vi "novasource_control.vi"(5 "Modulation Gain 2^i (i = -10 to 13)":i32 min=-10 max=13 step=1, 6 "Modulation On?":bool=TRUE, 7 "Frequency (1200-2000 MHz)":dbl=1251.451 min=1200.0 max=2000.0 step=0.001 format="%_7g") -> (0 "error out":errorcluster={"status"=FALSE, "code"=1073676294, "source"="VISA Read in novasource_control.vi"}, 1 "Locked?":bool=TRUE, 2 "RF State":bool=TRUE, 3 "Power":bool=TRUE)   [LabVIEW 2013]
uses:
  <vilib>/Instr/_visa.llb/VISA Configure Serial Port (Instr).vi
panel:
  in  "Case Constant\n(See Context Help)":i32
  out "Actual Gain":i32=1
  in  "Triggering Mode":u16(ring) items=["Continuous", "Momentary", "Toggle"]
  in  "Modulation Source":u16(ring)=1 items=["Internal Mod", "External Mod"]
  in  "Triggering Source":u16(ring) items=["Internal", "External"]
  in  "Attenuation Level (0-30)":i32 min=0 max=30 step=1
  in  "delay before read (ms)":u32=100
  in  "flow control":u16(ring) items=["None"=0, "XON/XOFF"=1, "RTS/CTS"=2, "DTR/DSR"=4]
  in  "stop bits":u16(ring)=10 items=["1.0"=10, "1.5"=15, "2.0"=20]
  in  "parity":u16(ring) items=["None", "Odd", "Even", "Mark", "Space"]
  in  "data bits":u16=8 min=5 max=8 step=1
  out "bytes read":u32=7
  in  "VISA resource name":refnum<visa-resource-name>="COM1"
  in  "baud rate":u32=38400
  # "Serial Settings"
  # "Nova Source Settings"
  # "Triggering"
  # "Modulation"
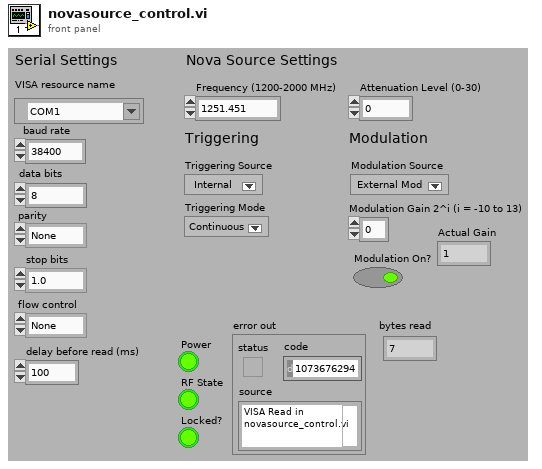
[diagram p1: front panel]
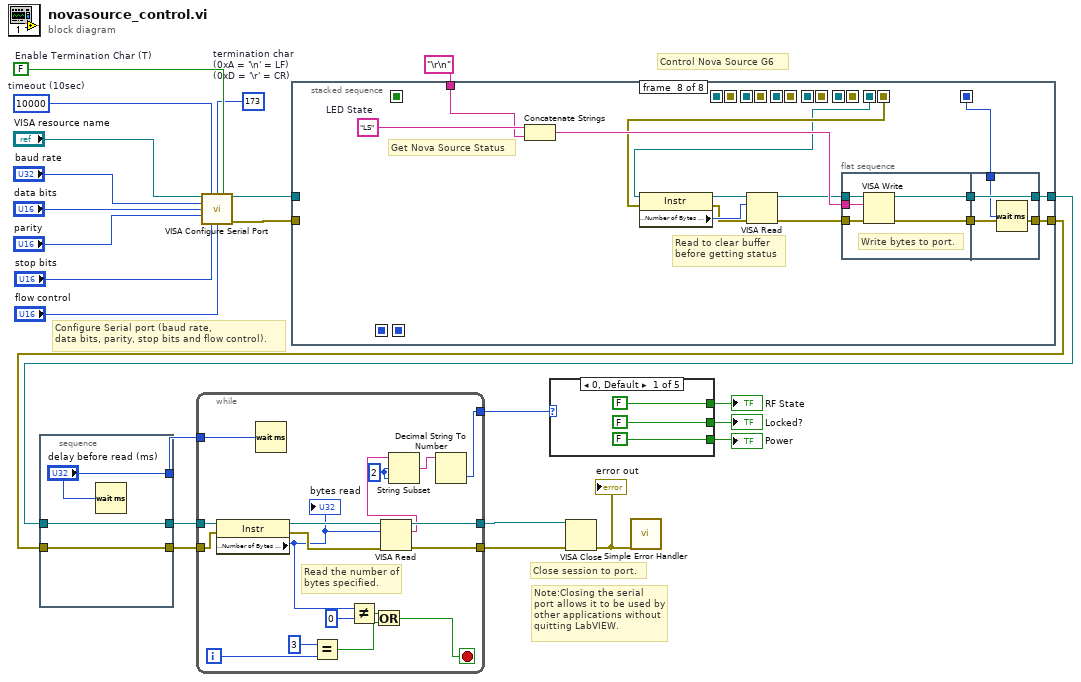
[diagram p0: block diagram]
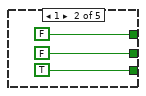
[diagram p2: hidden frame]
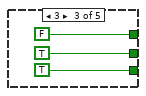
[diagram p3: hidden frame]
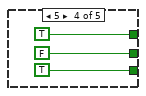
[diagram p4: hidden frame]
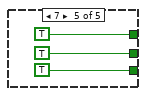
[diagram p5: hidden frame]
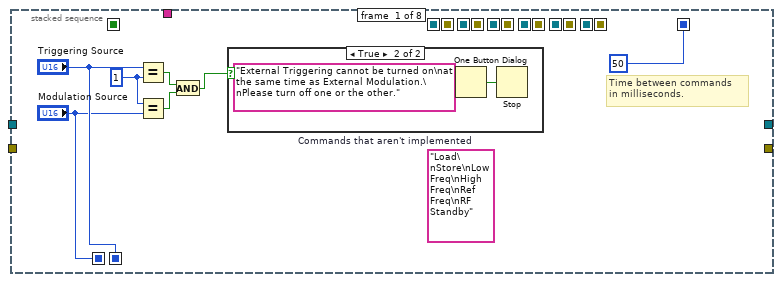
[diagram p6: hidden frame]
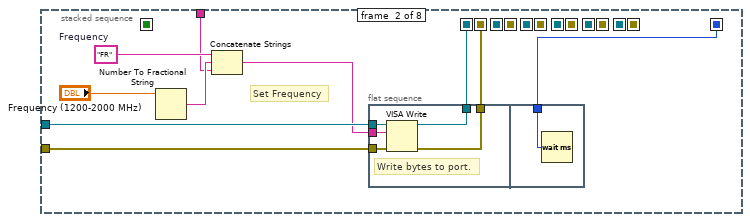
[diagram p8: hidden frame]
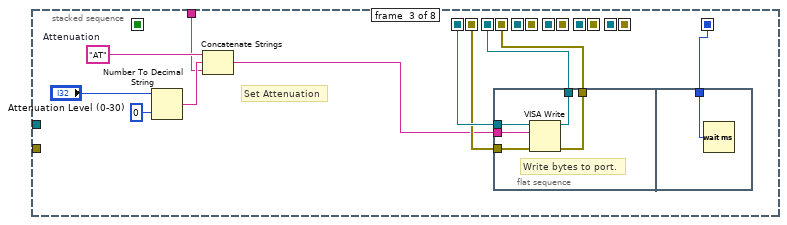
[diagram p9: hidden frame]
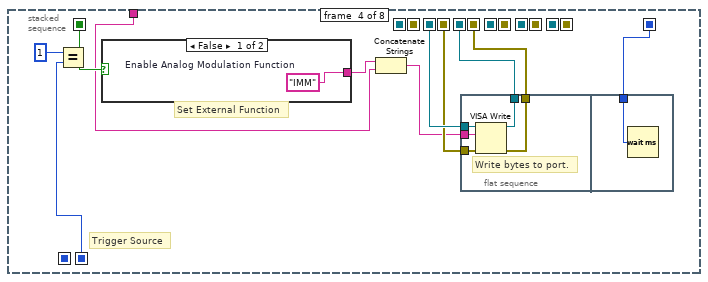
[diagram p10: hidden frame]
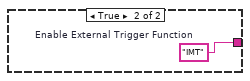
[diagram p11: hidden frame]
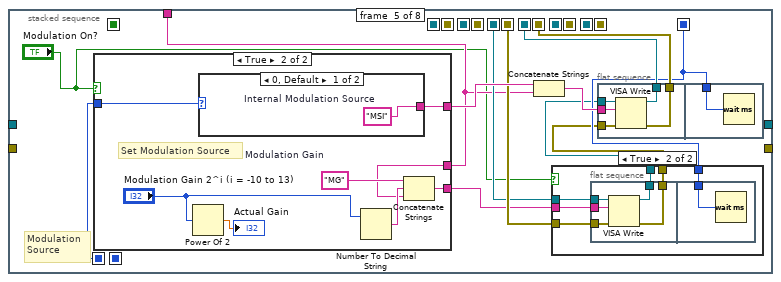
[diagram p12: hidden frame]
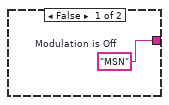
[diagram p14: hidden frame]
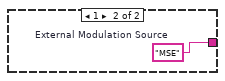
[diagram p15: hidden frame]
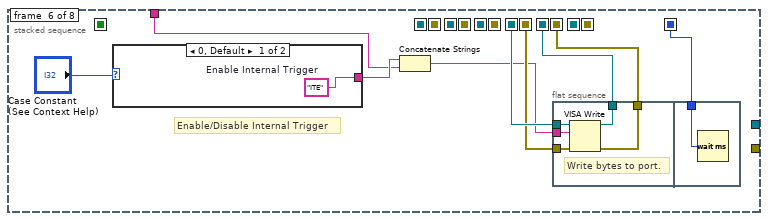
[diagram p16: hidden frame]
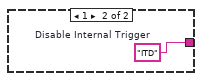
[diagram p17: hidden frame]
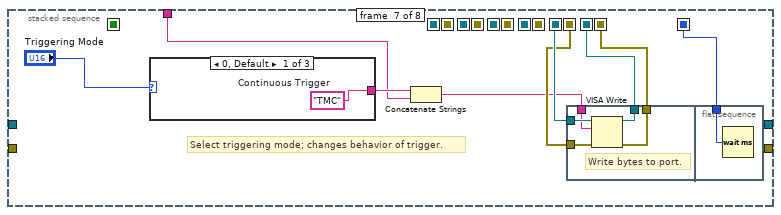
[diagram p18: hidden frame]
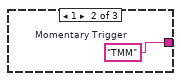
[diagram p19: hidden frame]
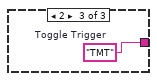
[diagram p20: hidden frame]
diagram:
  w10 = u8 173  # termination char (0xA = '\n' = LF) (0xD = '\r' = CR)
  w17 = FALSE  # Enable Termination Char (T)
  w18 = u32 10000  # timeout (10sec)
  # "Control Nova Source G6"
  # "Note:Closing the serial port allows it to be used by other applications without\nquitting LabVIEW."
  # "Configure Serial port (baud rate,\ndata bits, parity, stop bits and flow control)."
  # "Close session to port."
  n1 = call-poly "VISA Configure Serial Port"("VISA resource name"="VISA resource name", "timeout (10sec)"=w18, "termination char\n(0xA = '\\n' = LF)"=w10, "Enable Termination\nChar (T)"=w17, "baud rate (9600)"="baud rate", "data bits (8)"="data bits", "parity (0:none)"="parity", "stop bits (10: 1 bit)"="stop bits", "flow control (0:none)"="flow control") -> ("VISA resource name out"=w9:refnum<visa-resource-name>, "error out"=w8:errorcluster)  [unwired: 5 in]
  n2 = stacked-sequence {
    seq-local: [_ w37 _ _ _ _ _ _] -> [_ _ w57 _ _ _ _ _]
    seq-local: [_ w36 _ _ _ _ _ _] -> [_ _ w56 _ _ _ _ _]
    seq-local: [_ _ w52 _ _ _ _ _] -> [_ _ _ w77 _ _ _ _]
    seq-local: [_ _ w51 _ _ _ _ _] -> [_ _ _ w76 _ _ _ _]
    seq-local: [_ _ _ w75 _ _ _ _] -> [_ _ _ _ w89 _ _ _]
    seq-local: [_ _ _ w74 _ _ _ _] -> [_ _ _ _ w90 _ _ _]
    seq-local: ["Modulation Source" _ _ _ _ _ _ _] -> [_ _ _ _ w98 _ _ _]
    seq-local: ["Triggering Source" _ _ _ _ _ _ _] -> [_ _ _ w73 _ _ _ _]
    seq-local: [_ _ _ _ w97 _ _ _] -> [_ _ _ _ _ w138 _ _]
    seq-local: [_ _ _ _ w96 _ _ _] -> [_ _ _ _ _ w137 _ _]
    seq-local: [_ _ _ w71 _ _ _ _] -> [_ _ _ _ _ _ _ _]
    seq-local: [_ _ _ _ _ w136 _ _] -> [_ _ _ _ _ _ w155 _]
    seq-local: [_ _ _ _ _ w131 _ _] -> [_ _ _ _ _ _ w154 _]
    seq-local: [_ _ _ _ _ _ w152 _] -> [_ _ _ _ _ _ _ w167]
    seq-local: [_ _ _ _ _ _ w151 _] -> [_ _ _ _ _ _ _ w168]
    seq-local: [50 _ _ _ _ _ _ _] -> [_ w34 w50 w67 w93 w130 w147 w172]
    tunnel: w9 -> [_ w43 _ _ _ _ _ _]
    tunnel: w8 -> [_ w42 _ _ _ _ _ _]
    tunnel: [_ _ _ _ _ _ _ w179] -> w6
    tunnel: [_ _ _ _ _ _ _ w178] -> w7
    tunnel: "\r\n" -> [_ w38 w55 w69 w88 w133 w148 w176]
    frame #0 {
      (unwired) "Load\nStore\nLow Freq\nHigh Freq\nRef Freq\nRF Standby"  # Commands that aren't implemented
      w30 = u16 1 ("y")
      # "Time between commands\nin milliseconds."
      n3 = Equal?(x="Triggering Source", y=w30) -> (x = y?=w29:bool)
      n4 = Equal?(x=w30, y="Modulation Source") -> (x = y?=w31:bool)
      n5 = And(x=w29, y=w31) -> (x .and. y?=w28:bool)
      n6 = case shown="True" w28 {
        frame False {
        }
        frame True {
          n7 = One Button Dialog(message="External Triggering cannot be turned on\nat the same time as External Modulation.\nPlease turn off one or the other.") -> (true=w33:bool)  [unwired: 1 in]
          n8 = Stop(stop? (T)=w33) -> ()
        }
      }
    }
    frame #1 {
      w40 = "FR"  # Frequency
      # "Set Frequency"
      n9 = Number To Fractional String(number="Frequency (1200-2000 MHz)") -> (F-format string=w39:string)  [unwired: 3 in]
      n10 = Concatenate Strings(w40, w39, w38) -> (w35:string)
      n11 = flat-sequence {
        tunnel: w43 -> [w48]
        tunnel: w42 -> [w47]
        tunnel: [w46] -> w37
        tunnel: [w45] -> w36
        tunnel: w35 -> [w44]
        tunnel: w34 -> [w49]
        frame #0 {
          # "Write bytes to port."
          n12 = VISA Write(VISA resource name=w48, write buffer=w44, error in (no error)=w47) -> (VISA resource name out=w46:refnum<visa-resource-name>, error out=w45:errorcluster)  [unwired: 1 out]
        }
        frame #1 {
          n13 = Wait (ms)(milliseconds to wait=w49) -> ()  [unwired: 1 out]
        }
      }
    }
    frame #2 {
      w60 = "AT"  # Attenuation
      # "Set Attenuation"
      n14 = Number To Decimal String(number="Attenuation Level (0-30)", width (-)=i16 0) -> (decimal integer string=w58:string)
      n15 = Concatenate Strings(w60, w58, w55) -> (w53:string)
      n16 = flat-sequence {
        tunnel: w57 -> [w65]
        tunnel: w56 -> [w64]
        tunnel: w53 -> [w63]
        tunnel: [w62] -> w52
        tunnel: [w61] -> w51
        tunnel: w50 -> [w66]
        frame #0 {
          # "Write bytes to port."
          n17 = VISA Write(VISA resource name=w65, write buffer=w63, error in (no error)=w64) -> (VISA resource name out=w62:refnum<visa-resource-name>, error out=w61:errorcluster)  [unwired: 1 out]
        }
        frame #1 {
          n18 = Wait (ms)(milliseconds to wait=w66) -> ()  [unwired: 1 out]
        }
      }
    }
    frame #3 {
      # "Trigger Source"
      # "Set External Function"
      n19 = Equal?(x=u16 1, y=w73) -> (x = y?=w71:bool)
      n20 = case shown="False" w71 {
        tunnel: [w84 w85] -> w70
        frame False {
          w84 = "IMM"  # Enable Analog Modulation Function
        }
        frame True {
          w85 = "IMT"  # Enable External Trigger Function
        }
      }
      n21 = Concatenate Strings(w70, w69) -> (w68:string)
      n22 = flat-sequence {
        tunnel: w77 -> [w82]
        tunnel: w76 -> [w81]
        tunnel: [w80] -> w75
        tunnel: [w79] -> w74
        tunnel: w68 -> [w78]
        tunnel: w67 -> [w83]
        frame #0 {
          # "Write bytes to port."
          n23 = VISA Write(VISA resource name=w82, write buffer=w78, error in (no error)=w81) -> (VISA resource name out=w80:refnum<visa-resource-name>, error out=w79:errorcluster)  [unwired: 1 out]
        }
        frame #1 {
          n24 = Wait (ms)(milliseconds to wait=w83) -> ()  [unwired: 1 out]
        }
      }
    }
    frame #4 {
      # "Modulation\nSource"
      n25 = case shown="True" "Modulation On?" {
        tunnel: [w119 w127] -> w94
        tunnel: w98 -> [_ w126]
        tunnel: w88 -> [_ w121]
        tunnel: [_ w120] -> w86
        frame False {
          w119 = "MSN"  # Modulation is Off
        }
        frame True {
          w125 = "MG"  # Modulation Gain
          # "Set Modulation Source"
          n26 = Power Of 2(x="Modulation Gain 2^i (i = -10 to 13)") -> (2^x=→"Actual Gain":dbl)
          n27 = case shown="0, Default" w126 {
            tunnel: [w128 w129] -> w127
            frame 0, Default {
              w128 = "MSI"  # Internal Modulation Source
            }
            frame 1 {
              w129 = "MSE"  # External Modulation Source
            }
          }
          n28 = Number To Decimal String(number="Modulation Gain 2^i (i = -10 to 13)") -> (decimal integer string=w124:string)  [unwired: 1 in]
          n29 = Concatenate Strings(w125, w124, w121) -> (w120:string)
        }
      }
      n30 = Concatenate Strings(w94, w88) -> (w95:string)
      n31 = case shown="True" "Modulation On?" {
        tunnel: w93 -> [_ w106]
        tunnel: [w100 w105] -> w92
        tunnel: [w99 w104] -> w91
        tunnel: w90 -> [w99 w103]
        tunnel: w89 -> [w100 w102]
        tunnel: w86 -> [_ w101]
        frame False {
        }
        frame True {
          n32 = flat-sequence {
            tunnel: w102 -> [w111]
            tunnel: w103 -> [w110]
            tunnel: [w109] -> w105
            tunnel: w101 -> [w108]
            tunnel: [w107] -> w104
            tunnel: w106 -> [w112]
            frame #0 {
              n33 = VISA Write(VISA resource name=w111, write buffer=w108, error in (no error)=w110) -> (VISA resource name out=w109:refnum<visa-resource-name>, error out=w107:errorcluster)  [unwired: 1 out]
            }
            frame #1 {
              n34 = Wait (ms)(milliseconds to wait=w112) -> ()  [unwired: 1 out]
            }
          }
        }
      }
      n35 = flat-sequence {
        tunnel: w92 -> [w117]
        tunnel: w91 -> [w116]
        tunnel: [w115] -> w97
        tunnel: [w114] -> w96
        tunnel: w95 -> [w113]
        tunnel: w93 -> [w118]
        frame #0 {
          n36 = VISA Write(VISA resource name=w117, write buffer=w113, error in (no error)=w116) -> (VISA resource name out=w115:refnum<visa-resource-name>, error out=w114:errorcluster)  [unwired: 1 out]
        }
        frame #1 {
          n37 = Wait (ms)(milliseconds to wait=w118) -> ()  [unwired: 1 out]
        }
      }
    }
    frame #5 {
      # "Enable/Disable Internal Trigger"
      n38 = case shown="0, Default" "Case Constant\n(See Context Help)" {
        tunnel: [w145 w146] -> w135
        frame 0, Default {
          w145 = "ITE"  # Enable Internal Trigger
        }
        frame 1 {
          w146 = "ITD"  # Disable Internal Trigger
        }
      }
      n39 = Concatenate Strings(w135, w133) -> (w134:string)
      n40 = flat-sequence {
        tunnel: w138 -> [w143]
        tunnel: w137 -> [w142]
        tunnel: [w141] -> w136
        tunnel: w134 -> [w140]
        tunnel: [w139] -> w131
        tunnel: w130 -> [w144]
        frame #0 {
          # "Write bytes to port."
          n41 = VISA Write(VISA resource name=w143, write buffer=w140, error in (no error)=w142) -> (VISA resource name out=w141:refnum<visa-resource-name>, error out=w139:errorcluster)  [unwired: 1 out]
        }
        frame #1 {
          n42 = Wait (ms)(milliseconds to wait=w144) -> ()  [unwired: 1 out]
        }
      }
    }
    frame #6 {
      # "Select triggering mode; changes behavior of trigger."
      n43 = case shown="0, Default" "Triggering Mode" {
        tunnel: [w162 w163 w164] -> w150
        frame 0, Default {
          w162 = "TMC"  # Continuous Trigger
        }
        frame 1 {
          w163 = "TMM"  # Momentary Trigger
        }
        frame 2 {
          w164 = "TMT"  # Toggle Trigger
        }
      }
      n44 = Concatenate Strings(w150, w148) -> (w149:string)
      n45 = flat-sequence {
        tunnel: w155 -> [w160]
        tunnel: w154 -> [w159]
        tunnel: [w158] -> w152
        tunnel: [w157] -> w151
        tunnel: w149 -> [w156]
        tunnel: w147 -> [w161]
        frame #0 {
          # "Write bytes to port."
          n46 = VISA Write(VISA resource name=w160, write buffer=w156, error in (no error)=w159) -> (VISA resource name out=w158:refnum<visa-resource-name>, error out=w157:errorcluster)  [unwired: 1 out]
        }
        frame #1 {
          n47 = Wait (ms)(milliseconds to wait=w161) -> ()  [unwired: 1 out]
        }
      }
    }
    frame #7 {
      w177 = "LS"  # LED State
      # "Read to clear buffer\nbefore getting status"
      # "Get Nova Source Status"
      n48 = Concatenate Strings(w177, w176) -> (w175:string)
      n49 = property class="Instr"(reference=w167, error in=w168) -> (reference out=w170:refnum<visa-resource-name>, error out=w169:errorcluster, "Serial Settings:Number of Bytes at Serial Port"=w171:u32)
      n50 = VISA Read(VISA resource name=w170, byte count=w171, error in (no error)=w169) -> (VISA resource name out=w166:refnum<visa-resource-name>, error out=w165:errorcluster)  [unwired: 2 out]
      n51 = flat-sequence {
        tunnel: w166 -> [w182]
        tunnel: w165 -> [w181]
        tunnel: w175 -> [w180]
        tunnel: [w184] -> w174
        tunnel: [w183] -> w173
        tunnel: [w186] -> w178
        tunnel: [w187] -> w179
        tunnel: w174 -> [w187]
        tunnel: w173 -> [w186]
        tunnel: w172 -> [w185]
        frame #0 {
          # "Write bytes to port."
          n52 = VISA Write(VISA resource name=w182, write buffer=w180, error in (no error)=w181) -> (VISA resource name out=w184:refnum<visa-resource-name>, error out=w183:errorcluster)  [unwired: 1 out]
        }
        frame #1 {
          n53 = Wait (ms)(milliseconds to wait=w185) -> ()  [unwired: 1 out]
        }
      }
    }
  }
  n54 = stacked-sequence {
    tunnel: w7 -> [w190]
    tunnel: [w190] -> w13
    tunnel: w6 -> [w189]
    tunnel: [w189] -> w12
    tunnel: ["delay before read (ms)"] -> w11
    frame #0 {
      n55 = Wait (ms)(milliseconds to wait="delay before read (ms)") -> ()  [unwired: 1 out]
    }
  }
  n56 = while {
    tunnel: [w208] -> w22
    tunnel: [w207] -> w21
    tunnel: w12 -> [w206]
    tunnel: w13 -> [w204]
    tunnel: w11 -> [w195]
    tunnel: [w194] -> w5
    i -> [w199]
    stop <- w196 stop-if-true
    w192 = 2 ("length (rest)")
    # "Read the number of bytes specified."
    n57 = property class="Instr"(reference=w206, error in=w204) -> (reference out=w205:refnum<visa-resource-name>, error out=w203:errorcluster, "Serial Settings:Number of Bytes at Serial Port"=w202:u32)
    "bytes read" <- w202
    n58 = Wait (ms)(milliseconds to wait=w195) -> ()  [unwired: 1 out]
    n59 = Equal?(x=3, y=w199) -> (x = y?=w197:bool)
    n60 = Not Equal?(x=w202, y=u32 0) -> (x != y?=w200:bool)
    n61 = Or(x=w200, y=w197) -> (x .or. y?=w196:bool)
    n62 = VISA Read(VISA resource name=w205, byte count=w202, error in (no error)=w203) -> (VISA resource name out=w207:refnum<visa-resource-name>, read buffer=w193:string, error out=w208:errorcluster)  [unwired: 1 out]
    n63 = String Subset(string=w193, offset (0)=w192, length (rest)=w192) -> (substring=w191:string)
    n64 = Decimal String To Number(string=w191) -> (number=w194:i32)  [unwired: 2 in, 1 out]
  }
  n65 = case shown="0, Default" w5 {
    tunnel: [FALSE FALSE FALSE TRUE TRUE] -> w4
    tunnel: [FALSE FALSE TRUE FALSE TRUE] -> w3
    tunnel: [FALSE TRUE TRUE TRUE TRUE] -> w2
    frame 0, Default {
    }
    frame 1 {
    }
    frame 3 {
    }
    frame 5 {
    }
    frame 7 {
    }
  }
  "RF State" <- w4
  "Locked?" <- w3
  "Power" <- w2
  n66 = VISA Close(VISA resource name=w21, error in (no error)=w22) -> (error out=w20:errorcluster)
  "error out" <- w20
  n67 = call <vilib>:"Simple Error Handler.vi"("error in (no error)"=w20) -> ()  [unwired: 4 in, 5 out]
